vi "Camera.vi"() -> ()   [LabVIEW 2021]
uses:
  <vilib>/userDefined/High Color/IMAQdx.ctl
  <vilib>/vision/Management.llb/Cast Image 2 Method.ctl
  <vilib>/vision/driver/IMAQdx.llb/IMAQdx Camera Control Mode.ctl
  <vilib>/vision/driver/IMAQdx.llb/IMAQdx Acquisition Mode.ctl
  <vilib>/vision/driver/IMAQdx.llb/IMAQdx Buffer Number Mode.ctl
  <vilib>/vision/NI_Vision_Development_Module.lvlib
  <vilib>/vision/driver/NI_Vision_Acquisition_Software.lvlib
panel:
  in  "Session In":T1
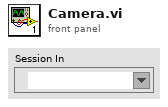
[diagram p1: front panel]
types:
  T1 = typedef "IMAQdx.ctl" = refnum<k21>
  T2 = typedef "NI_Vision_Acquisition_Software.lvlib/IMAQdx Buffer Number Mode.ctl" = enum32{"Next", "Last", "Buffer Number", "Every", "Last New"}
  T3 = typedef "NI_Vision_Acquisition_Software.lvlib/IMAQdx Acquisition Mode.ctl" = enum32{"One Shot", "Continuous"}
  T4 = typedef "NI_Vision_Acquisition_Software.lvlib/IMAQdx Camera Control Mode.ctl" = enum32{"Controller", "Listener"}
  T5 = typedef "Cast Image 2 Method.ctl" = u32
  T6 = typedef "Image Type" = u32
  T7 = typedef "IMAQ Image.ctl" = refnum<image>
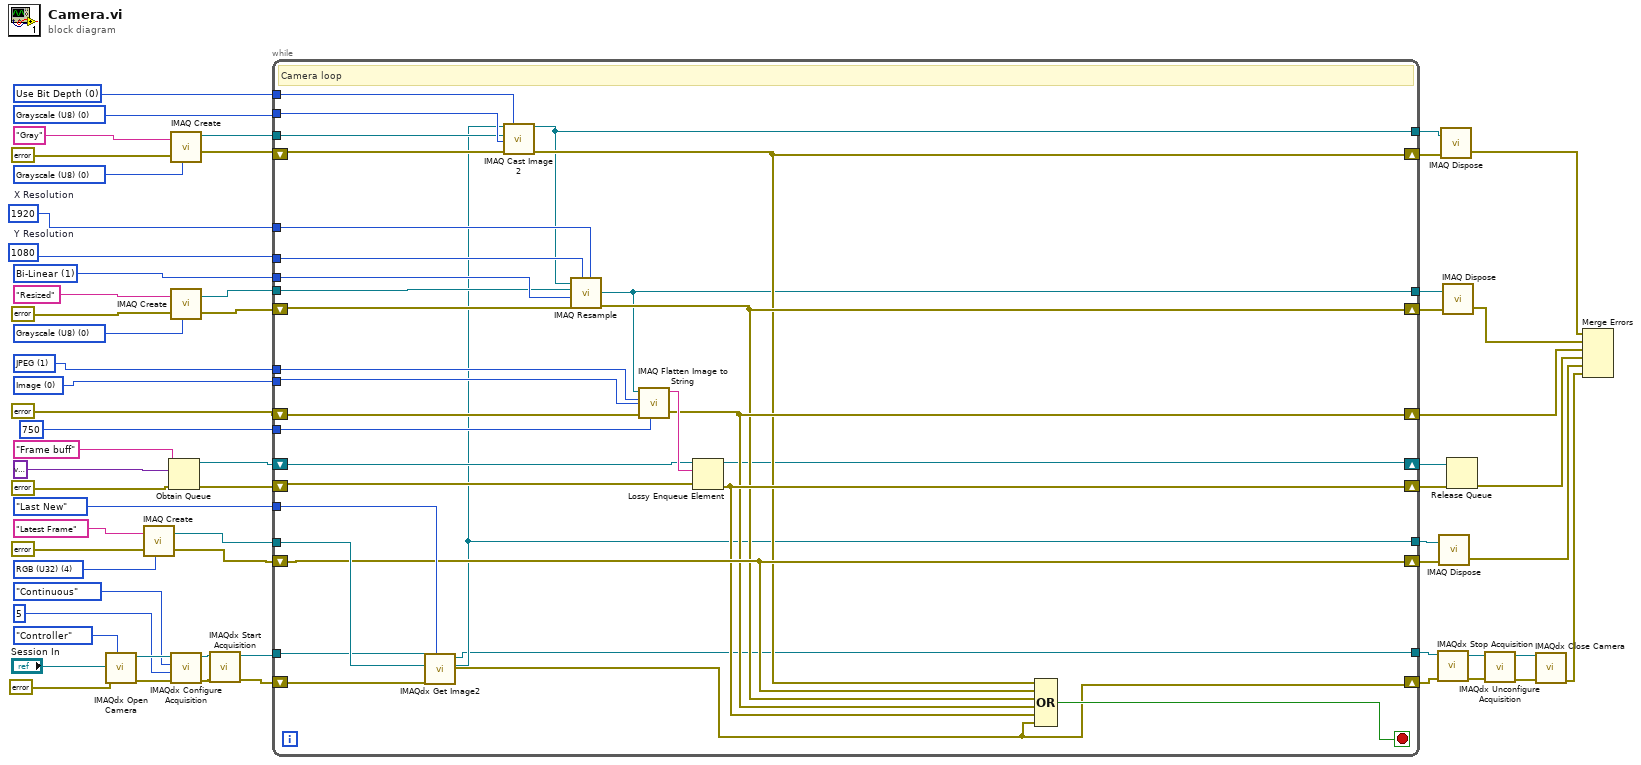
[diagram p0: block diagram]
diagram:
  w46 = 0 items=["Image", "Image and Vision Info", "Reference to Image"] ("Type of Flatten (Image and Vision Info)")
  w47 = 1 items=["None", "JPEG", "PACKED BINARY"] ("Compression (None)")
  w51 = u32 1 items=["Zero Order", "Bi-Linear", "Quadratic", "Cubic Spline"] ("Interpolation Type")
  w52 = 1080  # Y Resolution
  w53 = 1920  # X Resolution
  w56 = T5 0 items=["Use Bit Depth", "Shift", "Use Lookup Table"] ("Method")
  w58 = T6 4 items=["Grayscale (U8)", "Grayscale (I16)", "Grayscale (SGL)", "Complex (CSG)", "RGB (U32)", "HSL (U32)", "RGB (U64)", "Grayscale (U16)"] ("Image Type")
  w59 = T6 0 items=["Grayscale (U8)", "Grayscale (I16)", "Grayscale (SGL)", "Complex (CSG)", "RGB (U32)", "HSL (U32)", "RGB (U64)", "Grayscale (U16)"] ("Image Type")
  w57 = T6 0 items=["Grayscale (U8)", "Grayscale (I16)", "Grayscale (SGL)", "Complex (CSG)", "RGB (U32)", "HSL (U32)", "RGB (U64)", "Grayscale (U16)"] ("Image Type")
  w60 = T6 0 items=["Grayscale (U8)", "Grayscale (I16)", "Grayscale (SGL)", "Complex (CSG)", "RGB (U32)", "HSL (U32)", "RGB (U64)", "Grayscale (U16)"] ("Image Type")
  n1 = call <vilib>:"IMAQdx Open Camera.vi"("Camera Control Mode"=IMAQdx_Camera_Control_Mode."Controller", "error in"=errorcluster {"status"=FALSE, "code"=0, "source"=""}, "Session In"="Session In") -> ("error out"=w44:errorcluster, "Session Out"=w40:T1)  [unwired: 7 in]
  n2 = call "IMAQ Create"("Image Name"="Latest Frame", "Image Type"=w58, "error in (no error)"=errorcluster {"status"=FALSE, "code"=0, "source"=""} ("error in")) -> ("New Image"=w25:T7, "error out"=w22:errorcluster)  [unwired: 2 in]
  n3 = Obtain Queue(name (unnamed)="Frame buff", element data type=variant, error in (no error)=errorcluster {"status"=FALSE, "code"=0, "source"=""} ("error in")) -> (queue out=w26:refnum<queue>, error out=w27:errorcluster)  [unwired: 2 in, 1 out]
  n4 = call "IMAQ Create"("Image Name"="Gray", "Image Type"=w60, "error in (no error)"=errorcluster {"status"=FALSE, "code"=0, "source"=""}) -> ("New Image"=w54:T7, "error out"=w55:errorcluster)  [unwired: 2 in]
  n5 = call "IMAQ Create"("Image Name"="Resized", "Image Type"=w59, "error in (no error)"=errorcluster {"status"=FALSE, "code"=0, "source"=""} ("error in")) -> ("New Image"=w49:T7, "error out"=w48:errorcluster)  [unwired: 2 in]
  n6 = call <vilib>:"IMAQdx Configure Acquisition.vi"("error in"=w44, "Number of Buffers"=u32 5, "Continuous?"=IMAQdx_Acquisition_Mode."Continuous", "Session In"=w40) -> ("error out"=w43:errorcluster, "Session Out"=w39:T1)  [unwired: 6 in]
  n7 = call <vilib>:"IMAQdx Start Acquisition.vi"("error in"=w43, "Session In"=w39) -> ("error out"=w42:errorcluster, "Session Out"=w24:T1)  [unwired: 8 in]
  n8 = while {
    shift-right: [w68] -> w16
    shift-left: w55 -> [w91]
    tunnel: w57 -> [w93]
    tunnel: w56 -> [w92]
    tunnel: w54 -> [w90]
    tunnel: w53 -> [w89]
    tunnel: w52 -> [w88]
    tunnel: w51 -> [w87]
    tunnel: w49 -> [w86]
    shift-right: [w69] -> w17
    shift-left: w48 -> [w84]
    shift-right: [w70] -> w4
    shift-left: errorcluster {"status"=FALSE, "code"=0, "source"=""} ("error in") -> [w83]
    tunnel: w47 -> [w82]
    tunnel: w46 -> [w81]
    tunnel: 750 ("Quality (750)") -> [w80]
    shift-right: [w64] -> w13
    shift-left: w42 -> [w79]
    shift-right: [w71] -> w21
    shift-left: w27 -> [w78]
    shift-right: [w67] -> w20
    shift-left: w26 -> [w77]
    tunnel: w25 -> [w76]
    tunnel: w24 -> [w75]
    tunnel: IMAQdx_Buffer_Number_Mode."Last New" ("Buffer Number Mode (Next)") -> [w74]
    shift-right: [w72] -> w19
    shift-left: w22 -> [w72]
    tunnel: [w63] -> w18
    tunnel: [w66] -> w15
    tunnel: [w65] -> w14
    tunnel: [w62] -> w8
    stop <- w73 stop-if-true
    # "Camera loop"
    n9 = call <vilib>:"IMAQdx Get Image2.vi"("Buffer Number Mode (Next)"=w74, "error in"=w79, "Image In"=w76, "Session In"=w75) -> ("error out"=w64:errorcluster, "Image Out"=w63:T7, "Session Out"=w62:T1)  [unwired: 4 in, 1 out]
    n10 = call "IMAQ Cast Image 2"("Image Src"=w63, "Method"=w92, "Image Dst"=w90, "Image Type"=w93, "error in (no error)"=w91) -> ("Image Dst Out"=w66:T7, "error out"=w68:errorcluster)  [unwired: 9 in]
    n11 = call "IMAQ Resample"("X Resolution"=w89, "Y Resolution"=w88, "error in (no error)"=w84, "Interpolation Type"=w87, "Image Dst"=w86, "Image Src"=w66) -> ("error out"=w69:errorcluster, "Image Dst Out"=w65:T7)  [unwired: 4 in]
    n12 = call "IMAQ Flatten Image to String"("Quality (750)"=w80, "error in (no error)"=w83, "Type of Flatten (Image and Vision Info)"=w81, "Compression (None)"=w82, "Image"=w65) -> ("error out"=w70:errorcluster, "Data String"=w85:string)  [unwired: 5 in]
    n13 = Lossy Enqueue Element(queue=w77, element=w85, error in (no error)=w78) -> (queue out=w67:refnum<queue>, error out=w71:errorcluster)  [unwired: 2 out]
    n14 = Compound Arithmetic op=OR(w68, w72, w69, w70, w71, w64) -> (w73:bool)
  }
  n15 = call <vilib>:"IMAQdx Stop Acquisition.vi"("error in"=w13, "Session In"=w8) -> ("error out"=w10:errorcluster, "Session Out"=w9:T1)  [unwired: 8 in]
  n16 = call "IMAQ Dispose"("Image"=w18, "error in (no error)"=w19) -> ("error out"=w6:errorcluster)  [unwired: 4 in]
  n17 = call "IMAQ Dispose"("Image"=w15, "error in (no error)"=w16) -> ("error out"=w2:errorcluster)  [unwired: 4 in]
  n18 = call "IMAQ Dispose"("Image"=w14, "error in (no error)"=w17) -> ("error out"=w3:errorcluster)  [unwired: 4 in]
  n19 = Release Queue(queue=w20, error in (no error)=w21) -> (error out=w5:errorcluster)  [unwired: 1 in, 2 out]
  n20 = call <vilib>:"IMAQdx Unconfigure Acquisition.vi"("error in"=w10, "Session In"=w9) -> ("error out"=w12:errorcluster, "Session Out"=w11:T1)  [unwired: 8 in]
  n21 = call <vilib>:"IMAQdx Close Camera.vi"("error in"=w12, "Session In"=w11) -> ("error out"=w7:errorcluster)  [unwired: 9 in]
  n22 = Merge Errors(w2, w3, w4, w5, w6, w7) -> ()  [unwired: 1 out]
